vi "Clean Up After Init Error.vi"(8 "error in":errorcluster, 9 "initialize and close session behavior":T1, 10 "session in":variant, 11 "session factory in":refnum<class "Session Factory.lvclass">) -> (0 "error out":errorcluster)   [LabVIEW 2020, in "MeasurementLink VISA.lvlib" / "Session Factory.lvclass"]
doc: "Closes the local session in the event that an error occurred while creating a set of sessions. If the session represents a remote session, <b>initialize and close session behavior</b> indicates whether the remote session was created or attached to when initializing the local session. The default implementation sends \"Create and Close\" or \"Attach and Detach\" respectively to the \"Close MeasurementLink Session\" VI."
uses:
  Session Factory.lvclass
  MeasurementLink Instrument/ISession Factory/Initialize and Close Session Behavior.ctl
  Session Factory.lvclass/Session Factory.ctl
  MeasurementLink Instrument/ISession Factory/ISession Factory.lvclass
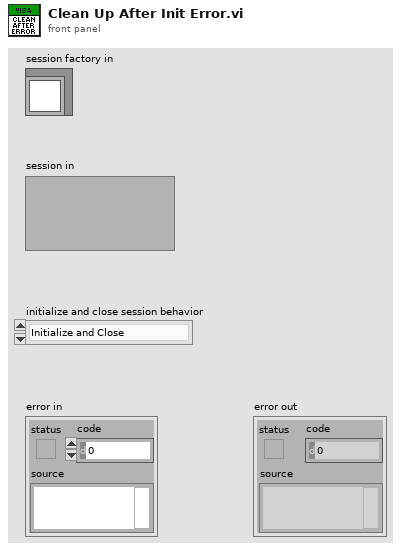
[diagram p1: front panel]
types:
  T1 = typedef "MeasurementLink Instrument.lvlib/ISession Factory.lvclass/Initialize and Close Session Behavior.ctl" = enum16{"Initialize and Close", "Attach and Detach", "Initialize and Detach", "Attach and Close"}
  T2 = typedef "MeasurementLink Instrument.lvlib/ISession Factory.lvclass/Remote Connection Options.ctl" = cluster{"session name":string, "address":string, "port":u32}
  T3 = typedef "MeasurementLink Instrument.lvlib/ISession Factory.lvclass/Session Initialization Parameters.ctl" = cluster{"resource name":string, "session name":string}
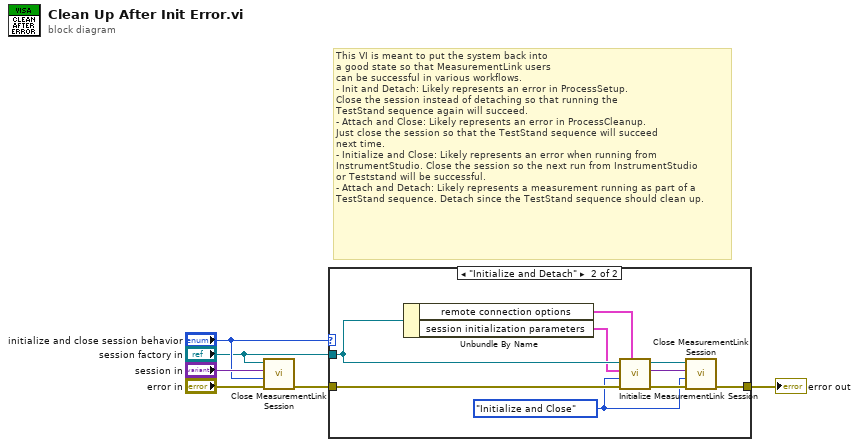
[diagram p0: block diagram]
diagram:
  # "This VI is meant to put the system back into\na good state so that MeasurementLink users\ncan be successful in various workflows.\n- Init and Detach: Likely represents an error in ProcessSetup.\nClose the session instead of detaching so that running the \nTestStand sequence again will succeed.\n- Attach and Close: Likely represents an error in ProcessCleanup.\nJust close the session so that the TestStand sequence will succeed\nnext time.\n- Initialize and Close: Likely represents an error when running from\nInstrumentStudio. Close the session so the next run from InstrumentStudio\nor Teststand will be successful.\n- Attach and Detach: Likely represents a measurement running as part of a\nTestStand sequence. Detach since the TestStand sequence should clean up."
  n1 = call-dynamic "Close MeasurementLink Session.vi"("error in"="error in", "initialize and close session behavior"="initialize and close session behavior", "session in"="session in", "session factory in"="session factory in") -> ("error out"=w3:errorcluster)  [unwired: 7 in]
  n2 = case shown="\"Initialize and Detach\"" "initialize and close session behavior" {
    tunnel: w3 -> [w7 w16]
    tunnel: "session factory in" -> [_ w10]
    tunnel: [w7 w14] -> w1
    frame "Initialize and Close", "Attach and Detach", "Attach and Close" {
    }
    frame "Initialize and Detach" {
      w12 = Initialize_and_Close_Session_Behavior."Initialize and Close" ("initialize and close session behavior")
      n3 = Unbundle By Name(w10) -> ("remote connection options"=w9:T2, "session initialization parameters"=w8:T3)
      n4 = call-dynamic "Initialize MeasurementLink Session.vi"("remote connection options"=w9, "error in"=w16, "initialize and close session behavior"=w12, "session initialization parameters"=w8, "session factory in"=w10) -> ("error out"=w15:errorcluster, "session out"=w13:variant, "session factory out"=w11:refnum<class "Session Factory.lvclass">)  [unwired: 4 in]
      n5 = call-dynamic "Close MeasurementLink Session.vi"("error in"=w15, "initialize and close session behavior"=w12, "session in"=w13, "session factory in"=w11) -> ("error out"=w14:errorcluster)  [unwired: 7 in]
    }
  }
  "error out" <- w1
